vi "Model - Get DB Current Step.vi"(8 "error in (no error)":errorcluster, 11 "View Model":T4) -> (0 "error out":errorcluster, 2 "Current Step Record":T1, 3 "View Model":T4)   [LabVIEW 2017]
doc: "Get actual DB Current Step Rules Value from DVR"
uses:
  Controls/View Model.ctl
  Controls/Shared Model.ctl
  Error Handler/Controls/Error Model.ctl
  Error Handler/Controls/Error Message.ctl
  Error Handler/Controls/Error Level.ctl
  Configuration/Controls/Database Model.ctl
  Configuration/Controls/Database Message.ctl
  Configuration/Controls/Database Command.ctl
  Configuration/Controls/Database Overhead.ctl
  Configuration/Controls/Database Status.ctl
  Configuration/Controls/Database Record.ctl
  Configuration/Controls/Database - Rule Record.ctl
  Controller/Controls/CNTRLR - Wash Step.ctl
  Controller/Controls/CNTRLR - Position.ctl
  Controller/Controls/CNTRLR - Model.ctl
  Controller/Controls/CNTRLR - Message.ctl
  Controller/Controls/CNTRLR - Command.ctl
  Controller/Controls/CNTRLR - Overhead.ctl
  Controller/Controls/CNTRLR - State.ctl
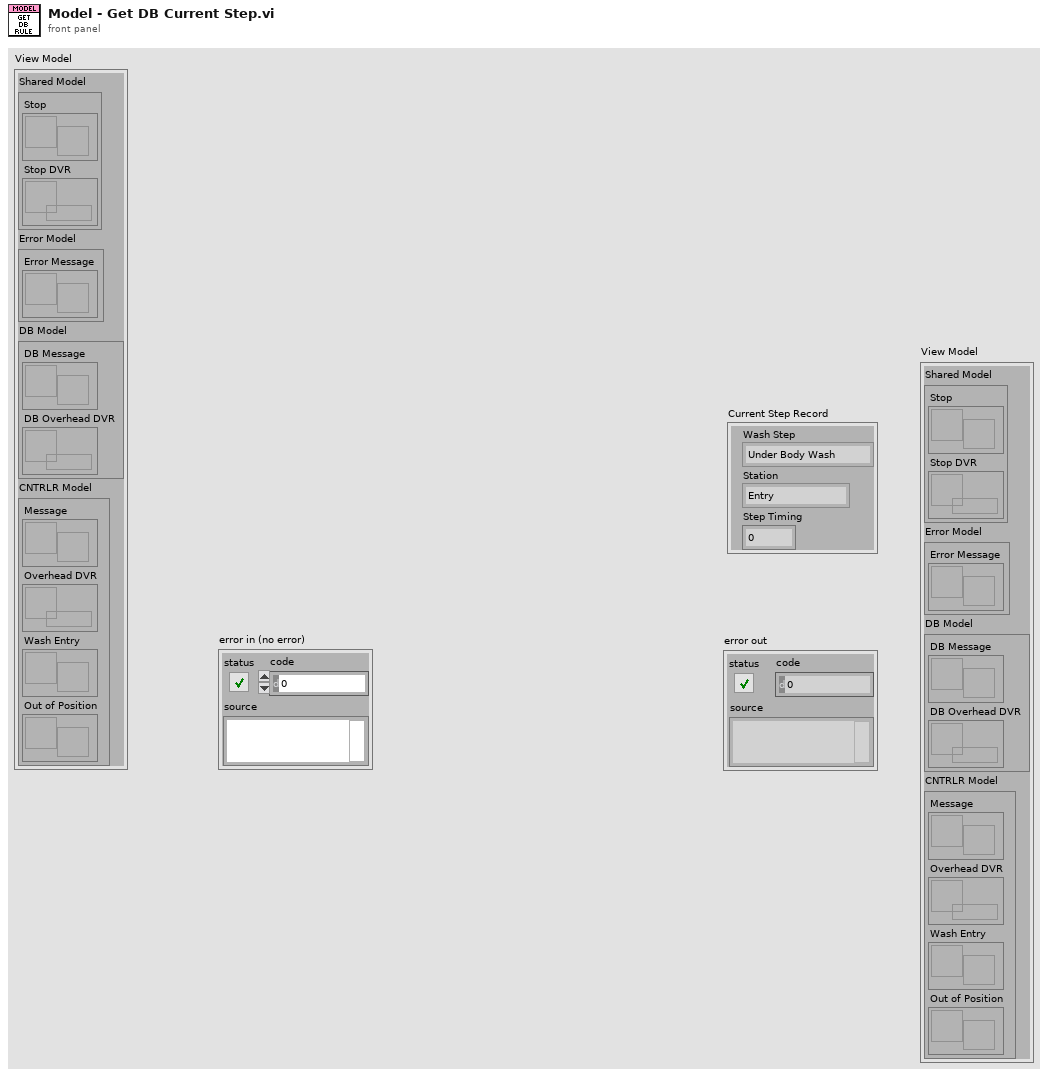
[diagram p1: front panel]
types:
  T1 = typedef "Database - Rule Record.ctl" = cluster{"Wash Step":T2, "Station":T3, "Step Timing":dbl}
  T2 = typedef "CNTRLR - Wash Step.ctl" = enum16{"Under Body Wash", "Bug Remover", "Pre-Soak", "High Pressure Wash", "Low Pressure Wax", "Spot Free Rinse", "Tire Shine Foam", "Air Dry", "None"}
  T3 = typedef "CNTRLR - Position.ctl" = enum16{"Entry", "Station 1", "Station 2", "Station 3", "Exit"}
  T4 = typedef "View Model.ctl" = cluster{"Shared Model":T5, "Error Model":T6, "DB Model":T7, "CNTRLR Model":T8}
  T5 = typedef "Shared Model.ctl" = cluster{"Stop":refnum<user-event>, "Stop DVR":refnum<data-value>}
  T6 = typedef "Error Model.ctl" = cluster{"Error Message":refnum<user-event>}
  T7 = typedef "Database Model.ctl" = cluster{"DB Message":refnum<user-event>, "DB Overhead DVR":refnum<data-value>}
  T8 = typedef "CNTRLR - Model.ctl" = cluster{"Message":refnum<user-event>, "Overhead DVR":refnum<data-value>, "Wash Entry":refnum<user-event>, "Out of Position":refnum<user-event>}
  T9 = typedef "Database Overhead.ctl" = cluster{"DB Status":T10, "DB Records":T11[], "Steps Rules":T1[], "Current Step Record":T1}
  T10 = typedef "Database Status.ctl" = enum16{"Unlocked", "Locked"}
  T11 = typedef "Database Record.ctl" = cluster{"Wash Step":string, "Station":string, "Step Duration":u32}
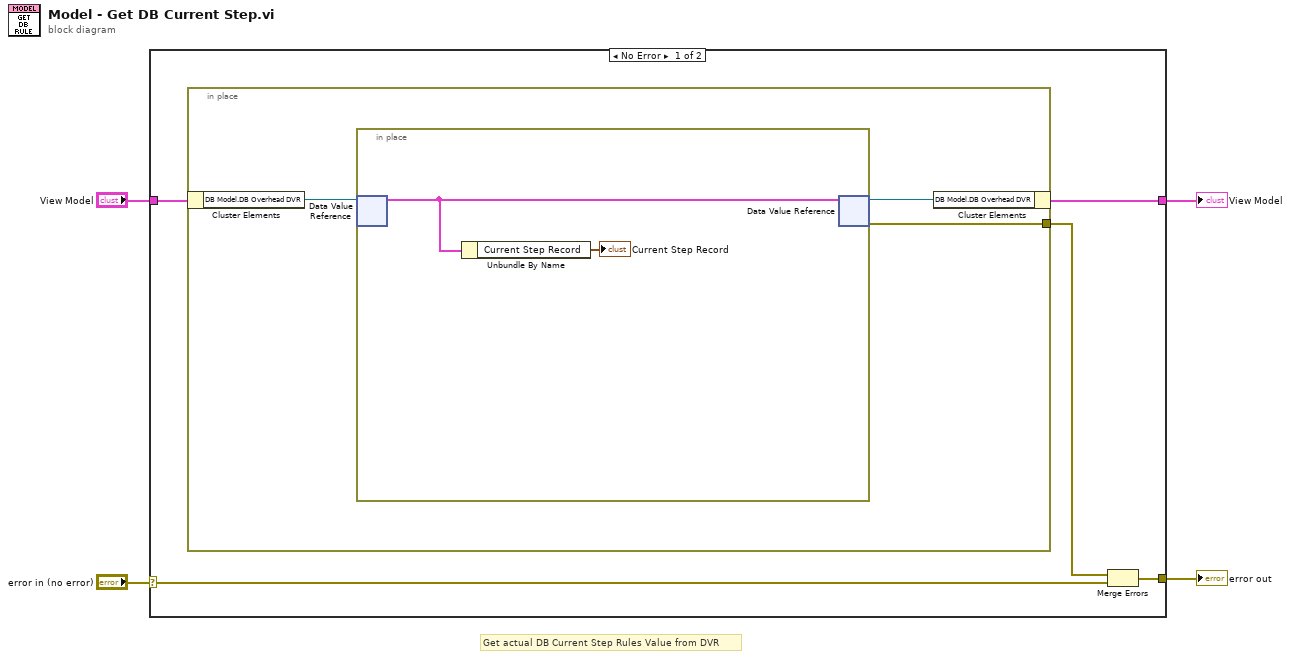
[diagram p0: block diagram]
diagram:
  # "Get actual DB Current Step Rules Value from DVR"
  n1 = case shown="No Error" "error in (no error)" {
    selector: "error in (no error)" -> [w7 w16]
    tunnel: [w5 w16] -> w3
    tunnel: "View Model" -> [w9 w15]
    tunnel: [w8 w15] -> w1
    frame No Error {
      n2 = in-place {
        in-place-border: [w10] -> w6
        n3 = in-place-cluster #1(w9) -> ("DB Model.DB Overhead DVR"=w12:refnum<data-value>)
        n4 = in-place {
          n5 = in-place-dvr #2(w12) -> (w14:T9)  [unwired: 1 out]
          n6 = Unbundle By Name(w14) -> ("Current Step Record"=→"Current Step Record":T1)
          n7 = in-place-dvr #2(w14) -> (w11:refnum<data-value>, w10:errorcluster)
        }
        n8 = in-place-cluster #1("DB Model.DB Overhead DVR"=w11) -> (w8:T4)
      }
      n9 = Merge Errors(w6, w7) -> (w5:errorcluster)
    }
    frame Error {
      # "If any Error occurred do nothing"
    }
  }
  "error out" <- w3
  "View Model" <- w1
